vi "main.vi"(10 "file path":path=path "C:/Users/DRX/Documents/Keysight/BenchVue/Test Flow/Exports/Flow 0.csv") -> (2 "file path 2":path=path "C:/Users/DRX/Desktop/IP/MEDIDAS/LAMINADA20.csv")   [LabVIEW 2021]
uses:
  <vilib>/Utility/file.llb/Write Delimited Spreadsheet (DBL).vi
panel:
  out "media tensao":dbl
  out "média cond":dbl
  out "condutividade":dbl[](array[numeric])
  out "voltagem":dbl[](array[numeric])
  out "sigma":dbl format="%#_13g"
  out "rho":dbl format="%#_13g"
  in  "i":dbl=0.1 format="%#_13g"
  in  "condutor?":bool
  in  "circular?":bool
  in  "s":dbl=0.001016
  in  "d":dbl=0.0222
  in  "w":dbl=0.0007
  in  "a":dbl=0.02055
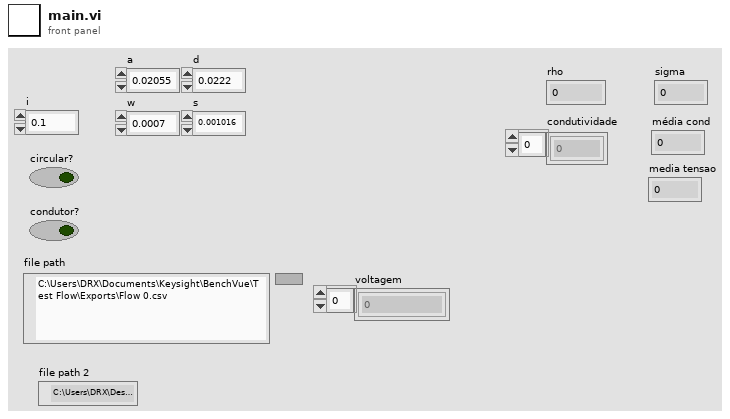
[diagram p1: front panel]
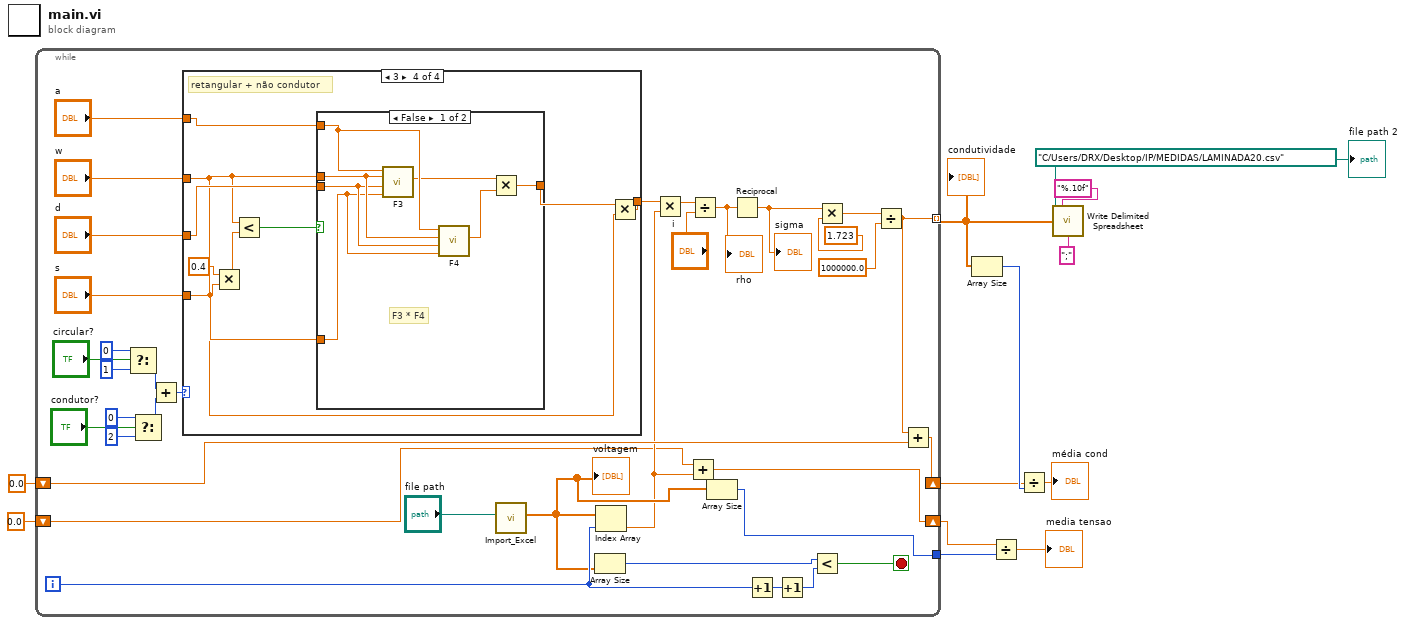
[diagram p0: block diagram]
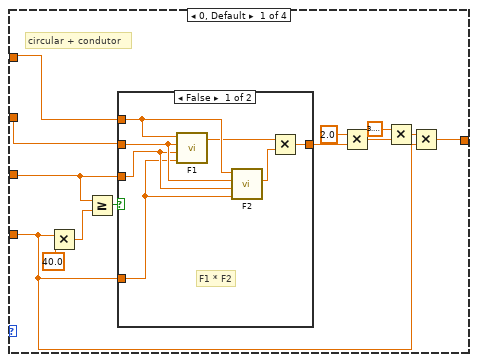
[diagram p2: hidden frame]
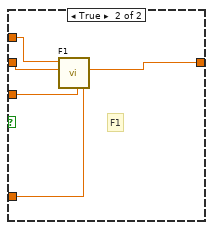
[diagram p3: hidden frame]
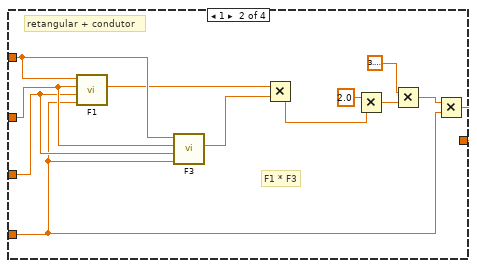
[diagram p4: hidden frame]
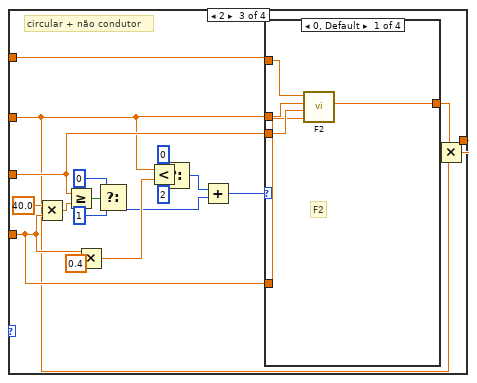
[diagram p5: hidden frame]
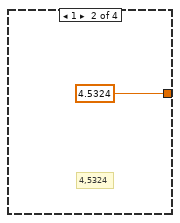
[diagram p6: hidden frame]
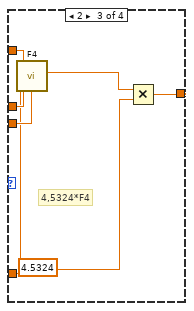
[diagram p7: hidden frame]
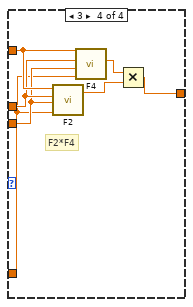
[diagram p8: hidden frame]
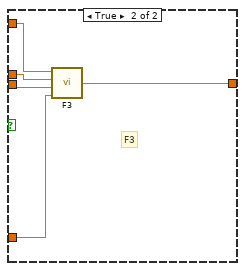
[diagram p9: hidden frame]
diagram:
  w8 = path "C:/Users/DRX/Desktop/IP/MEDIDAS/LAMINADA20.csv" ("file path")
  n1 = while {
    tunnel: [w20] -> w6 mode=indexing
    shift-right: [w18] -> w10
    shift-left: 0.0 -> [w19]
    shift-right: [w13] -> w3
    shift-left: 0.0 -> [w14]
    tunnel: [w16] -> w2
    i -> [w22]
    stop <- w25 stop-if-true
    n2 = Select(t=0, s="circular?", f=1) -> (s? t:f=w41:i32)
    n3 = Select(t=0, s="condutor?", f=2) -> (s? t:f=w40:i32)
    n4 = Add(x=w41, y=w40) -> (x+y=w39:i32)
    n5 = case shown="3" w39 {
      tunnel: "d" -> [w55 w82 w89 w128]
      tunnel: "w" -> [w56 w83 w86 w125]
      tunnel: "a" -> [w57 w84 w90 w129]
      tunnel: "s" -> [w49 w74 w88 w127]
      tunnel: [w48 w73 w85 w124] -> w34
      frame 0, Default {
        # "circular + condutor"
        n6 = Multiply(x=w49, y=40.0) -> (x*y=w60:dbl)
        n7 = Greater Or Equal?(x=w55, y=w60) -> (x >= y?=w58:bool)
        n8 = case shown="False" w58 {
          tunnel: w57 -> [w67 w72]
          tunnel: w56 -> [w66 w71]
          tunnel: w55 -> [w65 w70]
          tunnel: w49 -> [w64 w69]
          tunnel: [w61 w68] -> w54
          frame False {
            # "F1 * F2"
            n9 = call "F1.vi"("s"=w64, "d"=w65, "w"=w66, "a"=w67) -> ("F1"=w63:dbl)  [unwired: 7 in]
            n10 = call "F2.vi"("s"=w64, "d"=w65, "w"=w66, "a"=w67) -> ("F2"=w62:dbl)  [unwired: 7 in]
            n11 = Multiply(x=w63, y=w62) -> (x*y=w61:dbl)
          }
          frame True {
            # "F1"
            n12 = call "F1.vi"("s"=w69, "d"=w70, "w"=w71, "a"=w72) -> ("F1"=w68:dbl)  [unwired: 7 in]
          }
        }
        n13 = Multiply(x=2.0, y=w54) -> (x*y=w52:dbl)
        n14 = Multiply(x=3.141592653589793, y=w52) -> (x*y=w50:dbl)
        n15 = Multiply(x=w50, y=w49) -> (x*y=w48:dbl)
      }
      frame 1 {
        # "F1 * F3"
        # "retangular + condutor"
        n16 = call "F1.vi"("s"=w74, "d"=w82, "w"=w83, "a"=w84) -> ("F1"=w81:dbl)  [unwired: 7 in]
        n17 = call "F3.vi"("s"=w74, "d"=w82, "w"=w83, "a"=w84) -> ("F3"=w80:dbl)  [unwired: 7 in]
        n18 = Multiply(x=w81, y=w80) -> (x*y=w75:dbl)
        n19 = Multiply(x=2.0, y=w75) -> (x*y=w78:dbl)
        n20 = Multiply(x=3.141592653589793, y=w78) -> (x*y=w76:dbl)
        n21 = Multiply(x=w76, y=w74) -> (x*y=w73:dbl)
      }
      frame 2 {
        # "circular + não condutor"
        n22 = Multiply(x=40.0, y=w88) -> (x*y=w101:dbl)
        n23 = Greater Or Equal?(x=w89, y=w101) -> (x >= y?=w99:bool)
        n24 = Multiply(x=w88, y=0.4) -> (x*y=w103:dbl)
        n25 = Select(t=0, s=w99, f=1) -> (s? t:f=w92:i32)
        n26 = Less?(x=w86, y=w103) -> (x < y?=w96:bool)
        n27 = Select(t=0, s=w96, f=2) -> (s? t:f=w93:i32)
        n28 = Add(x=w93, y=w92) -> (x+y=w91:i32)
        n29 = case shown="0, Default" w91 {
          tunnel: w90 -> [w108 _ w114 w123]
          tunnel: w86 -> [w107 _ w113 w122]
          tunnel: w89 -> [w106 _ w112 w121]
          tunnel: w88 -> [w105 _ w111 w120]
          tunnel: [w104 4.5324 w110 w117] -> w87
          frame 0, Default {
            # "F2"
            n30 = call "F2.vi"("s"=w105, "d"=w106, "w"=w107, "a"=w108) -> ("F2"=w104:dbl)  [unwired: 7 in]
          }
          frame 1 {
            # "4,5324"
          }
          frame 2 {
            # "4,5324*F4"
            n31 = call "F4.vi"("s"=w111, "d"=w112, "w"=w113, "a"=w114) -> ("F4"=w115:dbl)  [unwired: 7 in]
            n32 = Multiply(x=w115, y=4.5324) -> (x*y=w110:dbl)
          }
          frame 3 {
            # "F2*F4"
            n33 = call "F2.vi"("s"=w120, "d"=w121, "w"=w122, "a"=w123) -> ("F2"=w118:dbl)  [unwired: 7 in]
            n34 = call "F4.vi"("s"=w120, "d"=w121, "w"=w122, "a"=w123) -> ("F4"=w119:dbl)  [unwired: 7 in]
            n35 = Multiply(x=w119, y=w118) -> (x*y=w117:dbl)
          }
        }
        n36 = Multiply(x=w87, y=w86) -> (x*y=w85:dbl)
      }
      frame 3 {
        # "retangular + não condutor"
        n37 = Multiply(x=0.4, y=w127) -> (x*y=w131:dbl)
        n38 = Less?(x=w125, y=w131) -> (x < y?=w130:bool)
        n39 = case shown="False" w130 {
          tunnel: w129 -> [w139 w144]
          tunnel: w125 -> [w138 w143]
          tunnel: w128 -> [w137 w142]
          tunnel: w127 -> [w136 w141]
          tunnel: [w133 w140] -> w126
          frame False {
            # "F3 * F4"
            n40 = call "F3.vi"("s"=w136, "d"=w137, "w"=w138, "a"=w139) -> ("F3"=w135:dbl)  [unwired: 7 in]
            n41 = call "F4.vi"("s"=w136, "d"=w137, "w"=w138, "a"=w139) -> ("F4"=w134:dbl)  [unwired: 7 in]
            n42 = Multiply(x=w135, y=w134) -> (x*y=w133:dbl)
          }
          frame True {
            # "F3"
            n43 = call "F3.vi"("s"=w141, "d"=w142, "w"=w143, "a"=w144) -> ("F3"=w140:dbl)  [unwired: 7 in]
          }
        }
        n44 = Multiply(x=w126, y=w125) -> (x*y=w124:dbl)
      }
    }
    n45 = call "Import_Excel.vi"("file path (dialog if empty)"="file path") -> ("voltagem"=w17:dbl[])  [unwired: 10 in]
    "voltagem" <- w17
    n46 = Array Size(array=w17) -> (size(s)=w24:i32)
    n47 = Index Array(array=w17, index=w22) -> (element=w15:dbl)
    n48 = Multiply(x=w34, y=w15) -> (x*y=w33:dbl)
    n49 = Add(x=w14, y=w15) -> (x+y=w13:dbl)
    n50 = Divide(x=w33, y="i") -> (x/y=w31:dbl)
    "rho" <- w31
    n51 = Array Size(array=w17) -> (size(s)=w16:i32)
    n52 = Reciprocal(x=w31) -> (1/x=w30:dbl)
    "sigma" <- w30
    n53 = Increment(x=w22) -> (x+1=w21:i32)
    n54 = Increment(x=w21) -> (x+1=w23:i32)
    n55 = Less?(x=w24, y=w23) -> (x < y?=w25:bool)
    n56 = Multiply(x=w30, y=1.723) -> (x*y=w28:dbl)
    n57 = Divide(x=w28, y=1000000.0) -> (x/y=w20:dbl)
    n58 = Add(x=w20, y=w19) -> (x+y=w18:dbl)
  }
  "condutividade" <- w6
  n59 = Array Size(array=w6) -> (size(s)=w11:i32)
  n60 = Divide(x=w3, y=w2) -> (x/y=→"media tensao":dbl)
  n61 = Divide(x=w10, y=w11) -> (x/y=→"média cond":dbl)
  n62 = call-poly <vilib>:"Write Delimited Spreadsheet.vi"("file path (dialog if empty)"=w8, "format (%.3f)"="%.10f", "1D data"=w6, "delimiter (\\t)"=";" ("delimiter (\\t)")) -> ()  [unwired: 10 in, 2 out]
  "file path 2" <- w8
